vi "AxisSttepsToGo.vi"() -> ()   [LabVIEW 2011]
panel:
  in  "Stack Axis Steps":dbl
  in  "Slow Axis Steps":dbl
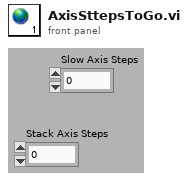
[diagram p1: front panel]
diagram:
